vi "Process Control Explorer.vi"() -> ()   [LabVIEW 2023]
doc: "Uses the Runge-Kutta 4th Order VI to determine and simulate the water flow through a tank based on the input flow, area of valve, and area of tank level equations as well as the initial water height."
uses:
  <vilib>/gmath/NI_Gmath.lvlib
panel:
  out "h(t)":T1(graph)
  out "time [s]":dbl=50.0
  in  "time end":dbl=50.0
  out "tank [cm]":dbl(slide)=50.0 scale=0.0..100.0
  in  "h0 [initial water height] [cm]":dbl=50.0
  in  "A [area of tank level] [cm^2]":dbl=20.0
  in  "a(t) [area of valve] [cm^2]":string="sin(t)+1"
  in  "fi(t) [input flow] [cm^3/sec]":string="340*square(t)"
  # "Overview: Uses the ODE Runge-Kutta 4th Order VI to determine and simulate the water flow through a tank based on the input flow, area of valve, and area of tank level equations as well as the initial water height.\nRequirements: LabVIEW Full Development System\nInstructions:\nRun the VI."
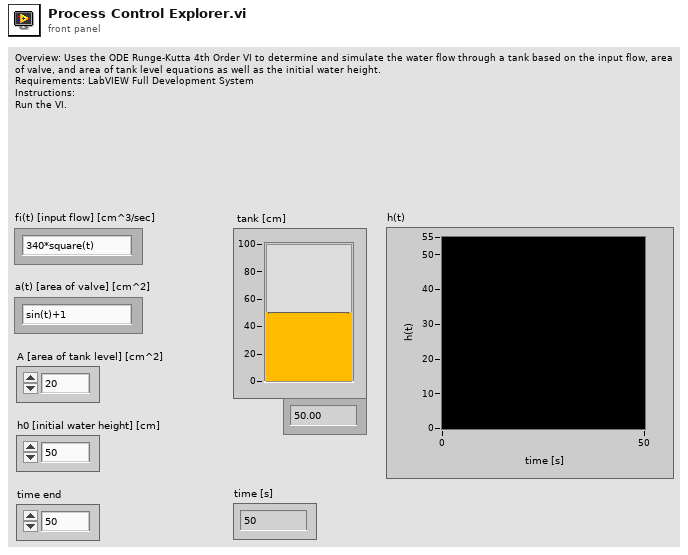
[diagram p1: front panel]
types:
  T1 = cluster{"Times":dbl[], "X Values (solution)":dbl[]}[]
  T2 = cluster{string, "a(t) [area of valve] [cm^2]":string}
  T3 = cluster{string, "fi(t) [input flow] [cm^3/sec]":string}
  T4 = cluster{string, "fi(t) [input flow] [cm^3/sec]":string}[]
  T5 = cluster{"Times":dbl[], "X Values (solution)":dbl[]}
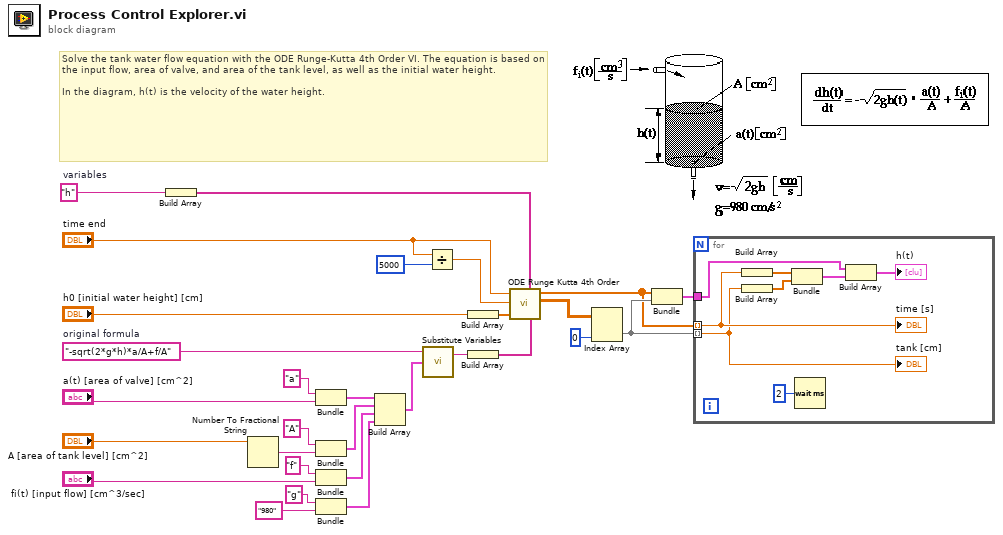
[diagram p0: block diagram]
diagram:
  w7 = "h"  # variables
  w23 = "-sqrt(2*g*h)*a/A+f/A"  # original formula
  # "Solve the tank water flow equation with the ODE Runge-Kutta 4th Order VI. The equation is based on the input flow, area of valve, and area of the tank level, as well as the initial water height.\n\nIn the diagram, h(t) is the velocity of the water height."
  n1 = Build Array(w7) -> (w6:string[])
  n2 = Number To Fractional String(number="A [area of tank level] [cm^2]") -> (F-format string=w16:string)  [unwired: 3 out]
  n3 = Bundle("a", "a(t) [area of valve] [cm^2]"="a(t) [area of valve] [cm^2]") -> (w12:T2)  [unwired: 1 in]
  n4 = Bundle("A", w16) -> (w13:cluster{string, string})  [unwired: 1 in]
  n5 = Bundle("f", "fi(t) [input flow] [cm^3/sec]"="fi(t) [input flow] [cm^3/sec]") -> (w11:T3)  [unwired: 1 in]
  n6 = Bundle("g", "980") -> (w1:cluster{string, string})  [unwired: 1 in]
  n7 = Build Array(w12, w13, w11, w1) -> (w10:T4)
  n8 = call <vilib>:"Substitute Variables.vi"("Substitution Rules"=w10, "original formula"=w23) -> ("formula after substitution"=w9:string)  [unwired: 1 in, 1 out]
  n9 = Divide(x="time end", y=5000) -> (x/y=w18:dbl)
  n10 = Build Array("h0 [initial water height] [cm]") -> (w22:dbl[])
  n11 = Build Array(w9) -> (w21:string[])
  n12 = call <vilib>:"ODE Runge Kutta 4th Order.vi"("time end"="time end", "h (step rate)"=w18, "X0"=w22, "X (name of variables)"=w6, "F(X,t) (right sides of the ODE\nas functions of X and t)"=w21) -> ("Times"=w4:dbl[], "X Values (solution)"=w20:dbl[][])  [unwired: 2 in, 2 out]
  n13 = Index Array(array=w20, index (col)=0) -> (element=w5:dbl[])  [unwired: 1 in]
  n14 = Bundle("Times"=w4, "X Values (solution)"=w5) -> (w29:T5)  [unwired: 1 out]
  n15 = for {
    tunnel: w29 -> [w31]
    tunnel: w4 -> [w33] mode=indexing
    tunnel: w5 -> [w32] mode=indexing
    n16 = Build Array(w33) -> (w34:dbl[])
    n17 = Build Array(w32) -> (w35:dbl[])
    n18 = Bundle(w34, w35) -> (w36:cluster{dbl[], dbl[]})  [unwired: 1 in]
    n19 = Wait (ms)(milliseconds to wait=u32 2) -> ()  [unwired: 1 out]
    n20 = Build Array(w31, w36) -> (→"h(t)":T1)
    "time [s]" <- w33
    "tank [cm]" <- w32
  }
